vi "AFG1022 Test.vi"() -> ()   [LabVIEW 2018]
doc: "Demonstrates how to configure then create an arbitrary waveform."
uses:
  C/Program Files (x86)/National Instruments/LabVIEW 2019/instr.lib/Tektronix AFG 1000 Series/Tektronix AFG 1000 Series.lvlib
panel:
  in  "Close Button":bool
  in  "Output Voltage, V":dbl(slide) scale=-10.0..10.0 scale format="%#.2g"
  in  "Channel (1: Channel 1)":u16(ring)=1 items=["Channel 1"=1, "Channel 2"=2]
  in  "Enable Output":bool
  in  "VISA resource name":refnum<visa-resource-name>
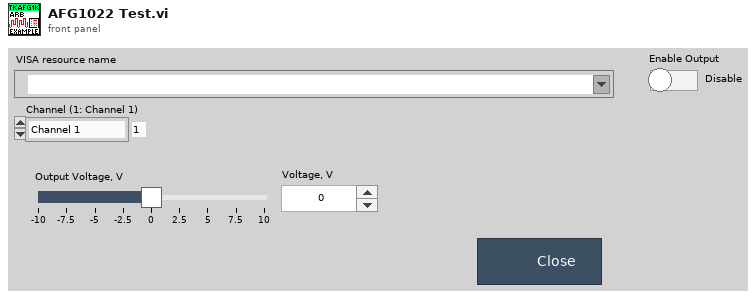
[diagram p1: front panel]
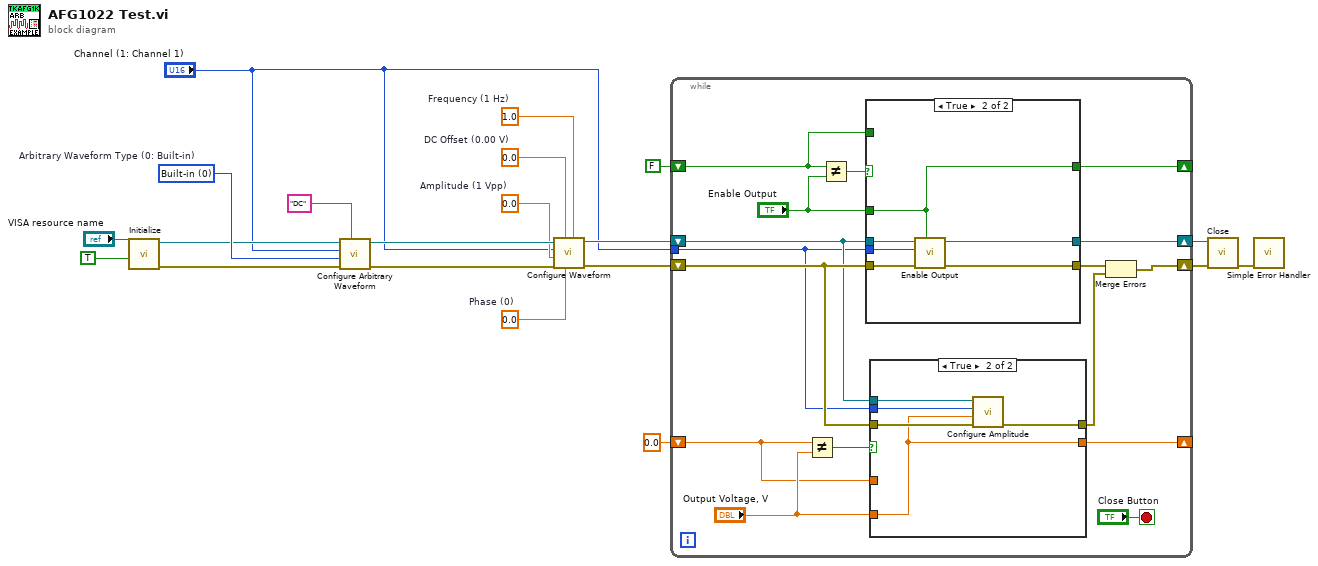
[diagram p0: block diagram]
diagram:
  w4 = 0.0  # Phase (0)
  w5 = 0.0  # Amplitude (1 Vpp)
  w6 = 1.0  # Frequency (1 Hz)
  w7 = 0.0  # DC Offset (0.00 V)
  w12 = u16 0 items=["Built-in", "User Waveform", "Edit Memory", "EFile"]  # Arbitrary Waveform Type (0: Built-in)
  n1 = call "Initialize.vi"("Reset (True)"=TRUE, "VISA resource name"="VISA resource name") -> ("error out"=w13:errorcluster, "VISA resource name out"=w11:refnum<visa-resource-name>)  [unwired: 8 in]
  n2 = call "Configure Arbitrary Waveform.vi"("Built-in Waveform Name (\"StairDown\")"="DC" ("Built-in Waveform Name (\"StairDown\")"), "error in (no error)"=w13, "Arbitrary Waveform Type (0: Built-in)"=w12, "Channel (1: Channel 1)"="Channel (1: Channel 1)", "VISA resource name"=w11) -> ("error out"=w8:errorcluster, "VISA resource name out"=w9:refnum<visa-resource-name>)  [unwired: 5 in]
  n3 = call "Configure Waveform.vi"("Frequency (1000 Hz)"=w6, "Phase (0)"=w4, "DC Offset (0.00 V)"=w7, "error in (no error)"=w8, "Amplitude (1 Vpp)"=w5, "Channel (1 Channel 1)"="Channel (1: Channel 1)", "VISA resource name"=w9) -> ("error out"=w3:errorcluster, "VISA resource name out"=w2:refnum<visa-resource-name>)  [unwired: 3 in]
  n4 = while {
    tunnel: "Channel (1: Channel 1)" -> [w24]
    shift-right: [w31] -> w16
    shift-left: w3 -> [w26]
    shift-right: [w36] -> w17
    shift-left: w2 -> [w25]
    shift-right: [w23] -> _
    shift-left: 0.0 -> [w22]
    shift-right: [w33] -> _
    shift-left: FALSE -> [w32]
    stop <- "Close Button" stop-if-true
    n5 = Not Equal?(x=w22, y="Output Voltage, V") -> (x != y?=w28:bool)
    n6 = Not Equal?(x=w32, y="Enable Output") -> (x != y?=w35:bool)
    n7 = case shown="True" w35 {
      tunnel: [w46 w52] -> w36
      tunnel: [w45 w51] -> w30
      tunnel: w26 -> [w45 w50]
      tunnel: w25 -> [w46 w49]
      tunnel: w24 -> [_ w48]
      tunnel: "Enable Output" -> [_ w47]
      tunnel: [w44 w47] -> w33
      tunnel: w32 -> [w44 _]
      frame False {
      }
      frame True {
        n8 = call "Enable Output.vi"("Enable Output (T: Enable)"=w47, "error in (no error)"=w50, "Channel (1: Channel 1)"=w48, "VISA resource name"=w49) -> ("error out"=w51:errorcluster, "VISA resource name out"=w52:refnum<visa-resource-name>)  [unwired: 6 in]
      }
    }
    n9 = case shown="True" w28 {
      tunnel: "Output Voltage, V" -> [_ w39]
      tunnel: w26 -> [w38 w43]
      tunnel: w25 -> [_ w42]
      tunnel: w24 -> [_ w41]
      tunnel: [w38 w40] -> w21
      tunnel: [w37 w39] -> w23
      tunnel: w22 -> [w37 _]
      frame False {
      }
      frame True {
        n10 = call "Configure Amplitude.vi"("error in (no error)"=w43, "Amplitude (1 Vpp)"=w39, "Channel (1 Channel 1)"=w41, "VISA resource name"=w42) -> ("error out"=w40:errorcluster)  [unwired: 6 in, 1 out]
      }
    }
    n11 = Merge Errors(w30, w21) -> (w31:errorcluster)
  }
  n12 = call "Close.vi"("error in (no error)"=w16, "VISA resource name"=w17) -> ("error out"=w20:errorcluster)  [unwired: 9 in]
  n13 = call <vilib>:"Simple Error Handler.vi"("error in (no error)"=w20) -> ()  [unwired: 4 in, 5 out]
